vi "Catapult Buttons unpack.vi"(9 "Jeffery's Buttons":T2, 10 "Jeffery's Axes":T1, 11 "Ian's Drive":T1) -> (1 "stop Catapult":bool, 2 "Arm Catapult":bool, 3 "Shoot":bool)   [LabVIEW 2013]
uses:
  <vilib>/Rock Robotics/WPI/Joystick/WPI_JoystickButtonState.ctl
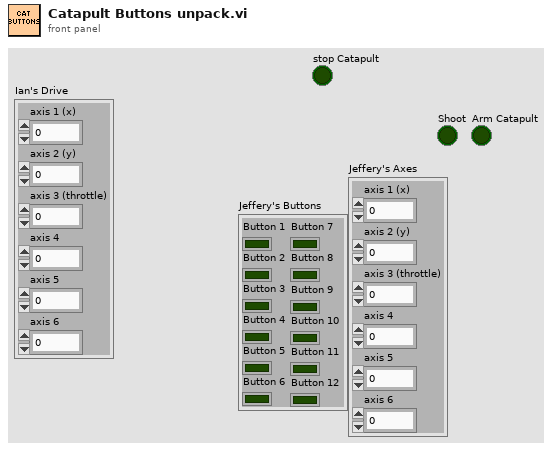
[diagram p1: front panel]
types:
  T1 = cluster{"axis 1 (x)":dbl, "axis 2 (y)":dbl, "axis 3 (throttle)":dbl, "axis 4":dbl, "axis 5":dbl, "axis 6":dbl}
  T2 = typedef "WPI_JoystickButtonState.ctl" = cluster{"Button 1":bool, "Button 2":bool, "Button 3":bool, "Button 4":bool, "Button 5":bool, "Button 6":bool, "Button 7":bool, "Button 8":bool, "Button 9":bool, "Button 10":bool, "Button 11":bool, "Button 12":bool}
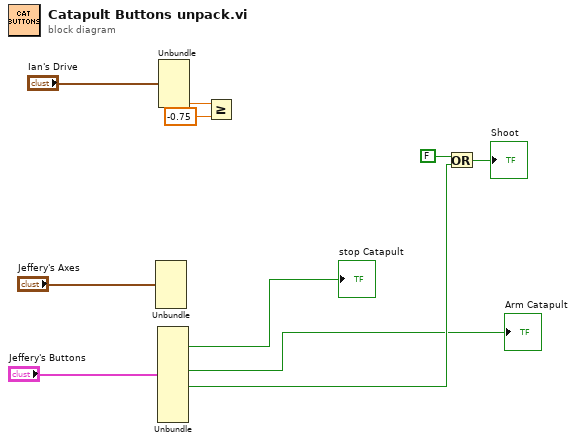
[diagram p0: block diagram]
diagram:
  n1 = Unbundle("Jeffery's Axes") -> ()  [unwired: 6 out]
  n2 = Unbundle("Jeffery's Buttons") -> ("Button 3"=→"stop Catapult":bool, "Button 6"=→"Arm Catapult":bool, "Button 8"=w5:bool)  [unwired: 9 out]
  n3 = Unbundle("Ian's Drive") -> ("axis 6"=w10:dbl)  [unwired: 5 out]
  n4 = Greater Or Equal?(x=w10, y=-0.75) -> ()  [unwired: 1 out]
  n5 = Or(x=FALSE, y=w5) -> (x .or. y?=→"Shoot":bool)
